vi "_testing.vi"() -> ()   [LabVIEW 2021]
panel:
  in  "Boolean":bool
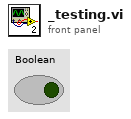
[diagram p1: front panel]
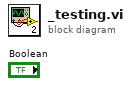
[diagram p0: block diagram]
diagram:
